vi "Haptic Device Test.vi"() -> ()   [LabVIEW 2013]
uses:
  Common/controls/Vector3D Fingers.ctl
  Common/classes/MF3/MF3.lvclass
  <vilib>/Platform/TimedLoop/XDataNode/timing_clust.ctl
  <vilib>/Platform/TimedLoop/XDataNode/nitl_modes.ctl
  <vilib>/Platform/TimedLoop/XDataNode/wakeup.ctl
  <userlib>/_matio/level5/Public/Write/Append Data Element.llb/Append Data Element (1D Array of Double).vi
  <userlib>/_matio/level5/Public/Write/Append Data Element.llb/Append Data Element (2D Array of Double).vi
  <vilib>/Platform/TimedLoop/XDataNode/XDataNode.xnode
  <userlib>/_matio/level5.lvlib
  <vilib>/Platform/TimedLoop/XDataNode/XDNodeRunTimeDep.lvlib
panel:
  in  "Finger Forces":T1={"Thumb"=[0.0, 0.0, 0.0], "Middle"=[0.0, 0.0, 0.0], "Index"=[0.0, 0.0, 0.0]}
  out "Current setpoints":dbl[](array[numeric]) format="%.2f"
  out "motor angles":dbl[](array[numeric]) format="%.2f"
  in  "MasterFinger":T2={"PID Gains"={"Proportional Gain"=20, "Integral Gain"=5, "Derivative Gain"=0}, "Current limit"=0.0} {"Current limit" min=0.0 max=1.0 step=0.1}
  in  "Data Logging":cluster{"Path":path, "Save":bool}={"Path"=path "c:/ni-rt/testing/grasping.mat", "Save"=TRUE}
  out "Logging Status":errorcluster
  out "MasterFinger Status":errorcluster
  in  "Stop":bool
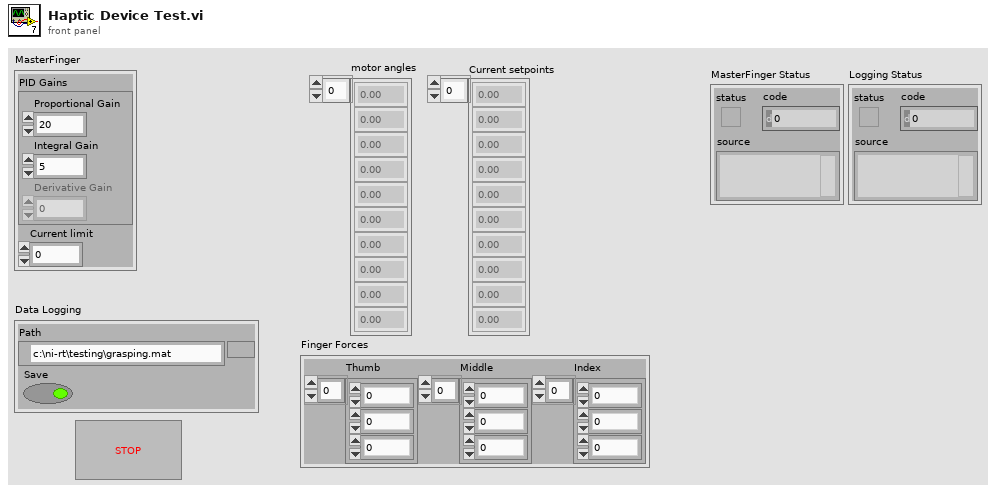
[diagram p1: front panel]
types:
  T1 = typedef "Vector3D Fingers.ctl" = cluster{"Thumb":dbl[], "Middle":dbl[], "Index":dbl[]}
  T2 = cluster{"PID Gains":cluster{"Proportional Gain":i16, "Integral Gain":i16, "Derivative Gain":i16}, "Current limit":dbl}
  T3 = cluster{"Proportional Gain":i16, "Integral Gain":i16, "Derivative Gain":i16}
  T4 = typedef "XDNodeRunTimeDep.lvlib/timing_clust.ctl" = cluster{"Expected End [f-1]":u64, "Actual End [f-1]":u64, "Finished Late? [f-1]":bool, "Expected End [i-1]":u64, "Actual End [i-1]":u64, "Finished Late? [i-1]":bool, "Expected Start [i]":u64, "Actual Start [i]":u64, "Expected Start [f]":u64, "Actual Start [f]":u64, "Source Name":string, "Structure Name":string, "Period":i64, "Deadline":i64, "Offset":i64, "Start":i64, "Priority":i32, "Timeout":i32, "Mode":T5, "Wakeup Reason":T6, "Error":errorcluster, "Source Type":string, "Secondary Source Type":string, "Global End Time":u64, "Global Start Time":u64, "Frame Duration":u64, "Iteration Duration":u64, "Assigned CPU":i32, "I/O Scan Engine Mode":u32}
  T5 = typedef "XDNodeRunTimeDep.lvlib/nitl_modes.ctl" = enum32{"No Change", "Process missed periods, maintain original phase", "Discard missed periods, maintain original phase", "Process missed periods, ignore original phase", "Discard missed periods, ignore original phase"}
  T6 = typedef "XDNodeRunTimeDep.lvlib/wakeup.ctl" = enum32{"Normal", "Aborted", "Asynchronous wakeup", "Timing source error", "Timed loop error", "Timeout"}
  T7 = enum16{"open", "replace", "create", "open or create", "replace or create", "replace or create with confirmation"}
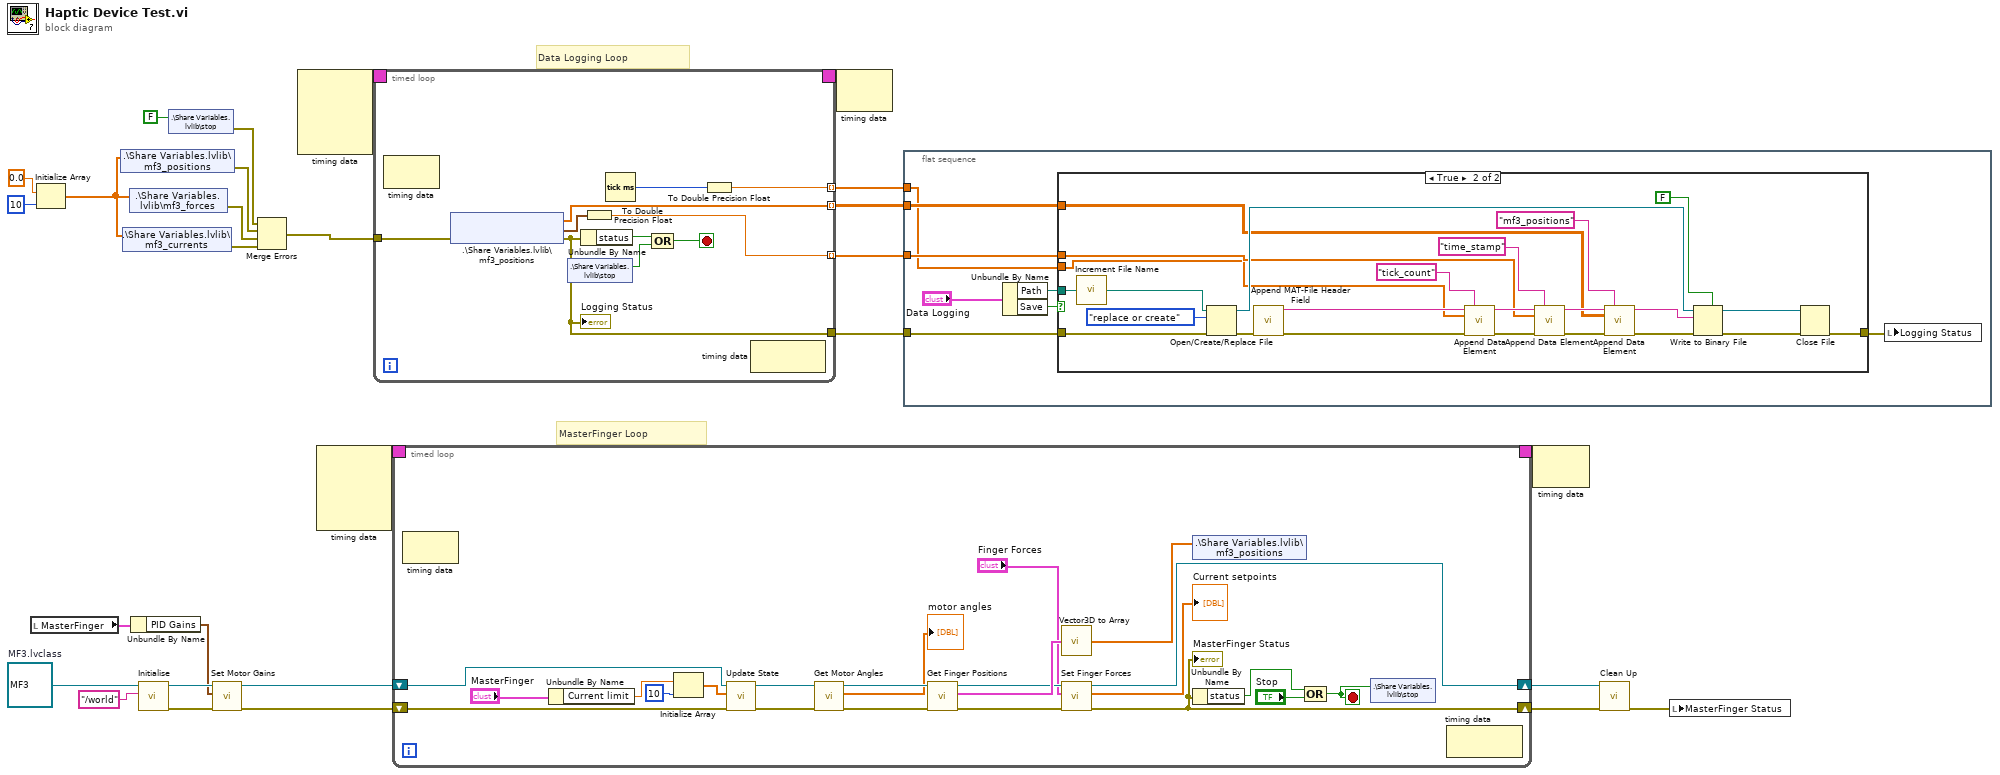
[diagram p0: block diagram]
diagram:
  w28 = refnum<class "MF3.lvclass"> refnum  # MF3.lvclass
  # "Data Logging Loop"
  # "MasterFinger Loop"
  n1 = local read "MasterFinger"() -> (w10:T2)
  n2 = Initialize Array "Initialize Array"(0.0 ("element"), 10 ("dimension size")) -> (w7:dbl[])
  n3 = shared-variable ".\\Share Variables.lvlib\\mf3_positions"(w7) -> (error out=w23:errorcluster)  [unwired: 1 in]
  n4 = shared-variable ".\\Share Variables.lvlib\\mf3_currents"(w7) -> (error out=w21:errorcluster)  [unwired: 1 in]
  n5 = shared-variable ".\\Share Variables.lvlib\\mf3_forces"(w7) -> (error out=w22:errorcluster)  [unwired: 1 in]
  n6 = Unbundle By Name(w10) -> ("PID Gains"=w9:T3)
  n7 = call "Initialise.vi"("frame"="/world", "MF3 in"=w28) -> ("error out"=w11:errorcluster, "MF3 out"=w12:refnum<class "MF3.lvclass">)  [unwired: 8 in]
  n8 = shared-variable ".\\Share Variables.lvlib\\stop"(FALSE ("stop")) -> (error out=w24:errorcluster)  [unwired: 1 in]
  n9 = call "Set Motor Gains.vi"("error in (no error)"=w11, "motor gains"=w9, "MF3 in"=w12) -> ("error out"=w1:errorcluster, "MF3 out"=w2:refnum<class "MF3.lvclass">)  [unwired: 7 in]
  n10 = Merge Errors(w24, w23, w22, w21) -> (w14:errorcluster)
  n11 = node-c288() -> (w4:T4)  [unwired: 4 in]
  n12 = node-c288() -> (w6:T4)  [unwired: 4 in]
  n13 = timed-loop {
    tunnel: [w34] -> w13
    tunnel: w14 -> [w38]
    tunnel: [w31] -> w17 mode=indexing
    tunnel: [w30] -> w16 mode=indexing
    tunnel: [w29] -> w15 mode=indexing
    timing: w4 -> [_]
    timing-out: [_] -> w3
    stop <- w35 stop-if-true
    n14 = node-c288() -> ()  [unwired: 1 in, 1 out]
    n15 = shared-variable ".\\Share Variables.lvlib\\mf3_positions"(error in=w38) -> (w31:dbl[], error out=w34:errorcluster, w32:timestamp)
    "Logging Status" <- w34
    n16 = shared-variable ".\\Share Variables.lvlib\\stop"() -> (w37:bool)  [unwired: 1 in, 1 out]
    n17 = Unbundle By Name(w34) -> ("status"=w36:bool)
    n18 = To Double Precision Float(number=w32) -> (double precision float=w30:dbl)
    n19 = Tick Count (ms)() -> (millisecond timer value=w33:u32)
    n20 = Compound Arithmetic op=OR(w36, w37) -> (w35:bool)
    n21 = To Double Precision Float(number=w33) -> (double precision float=w29:dbl)
    n22 = node-c288() -> ()  [unwired: 1 in, 1 out]
  }
  n23 = timed-loop {
    shift-right: [w44] -> w26
    shift-left: w2 -> [w52]
    shift-right: [w43] -> w20
    shift-left: w1 -> [w51]
    timing: w6 -> [_]
    timing-out: [_] -> w5
    stop <- w57 stop-if-true
    n24 = node-c288() -> ()  [unwired: 1 in, 1 out]
    n25 = Unbundle By Name("MasterFinger") -> ("Current limit"=w60:dbl)
    n26 = Initialize Array(w60, 10 ("dimension size")) -> (w58:dbl[])
    n27 = call "Update State.vi"("error in (no error)"=w51, "current_limits"=w58, "MF3 in"=w52) -> ("error out"=w49:errorcluster, "MF3 out"=w48:refnum<class "MF3.lvclass">)  [unwired: 7 in]
    n28 = call "Get Motor Angles.vi"("error in (no error)"=w49, "MF3 in"=w48) -> ("error out"=w47:errorcluster, "motor angles"=→"motor angles":dbl[], "MF3 out"=w50:refnum<class "MF3.lvclass">)  [unwired: 7 in]
    n29 = call "Get Finger Positions.vi"("error in (no error)"=w47, "MF3 in"=w50) -> ("error out"=w53:errorcluster, "Vector3D Fingers"=w55:T1, "MF3 out"=w54:refnum<class "MF3.lvclass">)  [unwired: 7 in]
    n30 = call "Vector3D to Array.vi"("Vector3D"=w55) -> ("Array"=w62:dbl[])
    n31 = call "Set Finger Forces.vi"("error in (no error)"=w53, "Finger Forces"="Finger Forces", "MF3 in"=w54) -> ("error out"=w43:errorcluster, "Current setpoints"=→"Current setpoints":dbl[], "MF3 out"=w44:refnum<class "MF3.lvclass">)  [unwired: 6 in]
    "MasterFinger Status" <- w43
    n32 = shared-variable ".\\Share Variables.lvlib\\mf3_positions"(w62) -> ()  [unwired: 1 in, 1 out]
    n33 = Unbundle By Name(w43) -> ("status"=w45:bool)
    n34 = Compound Arithmetic op=OR(w45, "Stop") -> (w57:bool)
    n35 = shared-variable ".\\Share Variables.lvlib\\stop"(w57) -> ()  [unwired: 1 in, 1 out]
    n36 = node-c288() -> ()  [unwired: 1 in, 1 out]
  }
  n37 = node-c288(w3) -> ()  [unwired: 1 out]
  n38 = flat-sequence {
    tunnel: w17 -> [w71]
    tunnel: w16 -> [w70]
    tunnel: w15 -> [w69]
    tunnel: w13 -> [w68]
    frame #0 {
      n39 = Unbundle By Name("Data Logging") -> ("Path"=w66:path, "Save"=w65:bool)
      n40 = case shown="True" w65 {
        tunnel: [w73 w82] -> w72
        tunnel: w71 -> [_ w81]
        tunnel: w70 -> [_ w80]
        tunnel: w69 -> [_ w79]
        tunnel: w68 -> [w73 w78]
        tunnel: w66 -> [_ w76]
        frame False {
        }
        frame True {
          n41 = call "Increment File Name.vi"("Full Path"=w76) -> ("New Path"=w83:path)
          n42 = Open/Create/Replace File(file path (use dialog)=w83, error in=w78, operation (0:open)=T7."replace or create") -> (refnum out=w84:refnum<file>, error out=w77:errorcluster)  [unwired: 3 in, 1 out]
          n43 = call <userlib>:"Append MAT-File Header Field.vi"("error"=w77) -> ("result string"=w93:string, "error out"=w92:errorcluster)  [unwired: 13 in]
          n44 = call-poly <userlib>:"Append Data Element.vi"("initial string"=w93, "Data Name"="tick_count", "data"=w79, "error in"=w92) -> ("result string"=w87:string, "error out"=w86:errorcluster)  [unwired: 10 in]
          n45 = call-poly <userlib>:"Append Data Element.vi"("initial string"=w87, "Data Name"="time_stamp", "data"=w80, "error in"=w86) -> ("result string"=w89:string, "error out"=w88:errorcluster)  [unwired: 10 in]
          n46 = call-poly <userlib>:"Append Data Element.vi"("initial string"=w89, "Data Name"="mf3_positions" ("array name"), "data"=w81, "error in"=w88) -> ("result string"=w75:string, "error out"=w74:errorcluster)  [unwired: 10 in]
          n47 = Write to Binary File(file (use dialog)=w84, data=w75, error in=w74, 5:FALSE ("prepend array or string size? (T)")) -> (refnum out=w95:refnum<file>, error out=w94:errorcluster)  [unwired: 2 in, 1 out]
          n48 = Close File(refnum=w95, error in=w94) -> (error out=w82:errorcluster)  [unwired: 1 out]
        }
      }
      n49 = local write "Logging Status"(w72) -> ()
    }
  }
  n50 = node-c288(w5) -> ()  [unwired: 1 out]
  n51 = call "Clean Up.vi"("error in (no error)"=w20, "MF3 in"=w26) -> ("error out"=w8:errorcluster)  [unwired: 8 in, 1 out]
  n52 = local write "MasterFinger Status"(w8) -> ()
